vi "Function.vi"(8 "error in (no error)":errorcluster, 10 "Value":i8, 11 "Two Terminal in":refnum<class "Decrement_I8.lvclass">) -> (0 "error out":errorcluster, 2 "Result":i8, 3 "Two Terminal out":refnum<class "Decrement_I8.lvclass">)   [LabVIEW 2021, in "Decrement_I8.lvclass"]
uses:
  Decrement_I8.lvclass
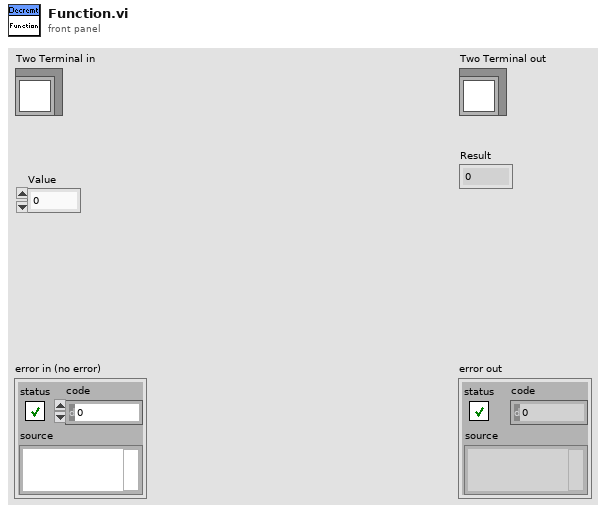
[diagram p1: front panel]
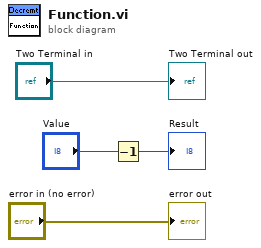
[diagram p0: block diagram]
diagram:
  n1 = Decrement(x="Value") -> (x-1=→"Result":i8)
  "error out" <- "error in (no error)"
  "Two Terminal out" <- "Two Terminal in"
